vi "Query Tidepool.vi"(8 "error in (no error)":errorcluster, 9 "Day":string, 10 "Starting Path":string, 11 "FTP Server":string) -> (0 "error out":errorcluster, 2 "dir list":T1[](array[typedef]), 3 "Total SBD Files In Dir":i32)   [LabVIEW 2014]
uses:
  <vilib>/FTP/ftp2.llb/FTP File Info.ctl
  <vilib>/FTP/NI_FTP.lvlib
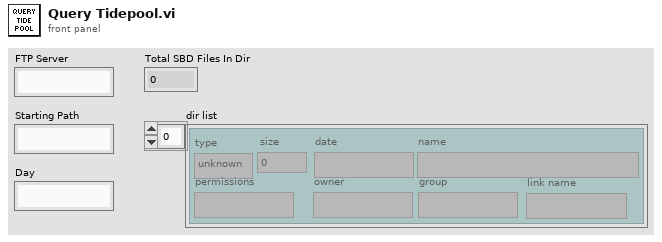
[diagram p1: front panel]
types:
  T1 = typedef "NI_FTP.lvlib/FTP File Info.ctl" = cluster{"type":enum16{"unknown", "file", "dir", "link"}, "permissions":string, "owner":string, "group":string, "size":i32, "date":string, "name":string, "link name":string}
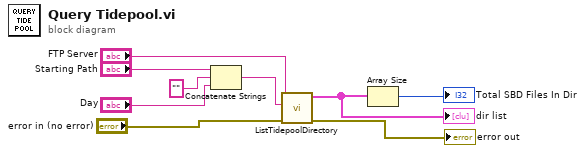
[diagram p0: block diagram]
diagram:
  n1 = Concatenate Strings("Starting Path", "" ("string"), "Day") -> (w4:string)
  n2 = call "ListTidepoolDirectory.vi"("error in (no error)"="error in (no error)", "Starting Path"=w4, "FTP Server"="FTP Server") -> ("error out"=→"error out":errorcluster, "dir list"=w6:T1[])  [unwired: 7 in]
  "dir list" <- w6
  n3 = Array Size(array=w6) -> (size(s)=→"Total SBD Files In Dir":i32)
